vi "Keys.vi"(11 "Dictionary in":variant) -> (0 "Keys":string[](array[string]), 3 "Dictionary out":variant)   [LabVIEW 2011, in "Dictionary.lvlib"]
doc: "Returns all keys in the dictionary."
uses:
  Dictionary.lvlib
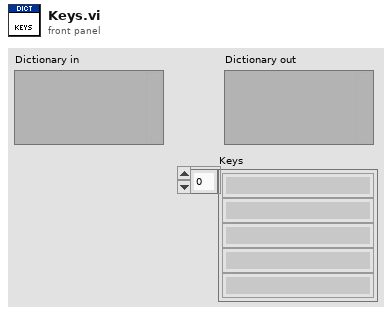
[diagram p1: front panel]
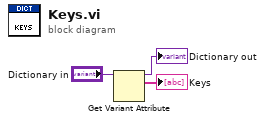
[diagram p0: block diagram]
diagram:
  n1 = Get Variant Attribute(Variant="Dictionary in") -> (duplicate Variant=→"Dictionary out":variant, names=→"Keys":string[])  [unwired: 3 in, 2 out]
